vi "Transmitter_SC.vi"() -> ()   [LabVIEW 2022 SP3]
uses:
  <instrlib>/niUSRP/niUSRP Write Tx Data (CDB Cluster).vi
panel:
  in  "Alpha":dbl(slide)=0.17500000000000002 step=0.005 scale=0.0..1.0
  in  "Tab Control":enum32{"USRP Parameters", "Transmission"}(tab)
  in  "USRP ControledParameters 2":T1={"Active Antenna"="TX1", "Gain (dB)"=0.0, "Carrier Frequency"=2400000000.0, "IQ Rate"=2000000.0, "Active Channel"="0"} {"IQ Rate" format="%#_6p"; "Carrier Frequency" format="%#_6p"; "Gain (dB)" format="%#_6f"}
  in  "Device selection":refnum<k15>="RIO0"
  in  "stop":bool
  out "Error out":errorcluster
  in  "Modulation parameter":T2
  out "Bits length":i32
  out "Bits length 2":i32
  out "Frame Duration":dbl format="%#_6p"
  out "Coerced Parameters":T3={"IQ Rate"=100000.0, "Carrier  Freq."=100000.0, "Gain"=0.0} {"Gain" format="%#_6f"; "Carrier  Freq." format="%#_6p"; "IQ Rate" format="%#_6p"}
  out "Transmitted Waveform":cluster{"t0":dbl, "dt":dbl, "Y":dbl[]}(graph)
  in  "Message 2":string="ptua. At vero eos et accusam et justo duo dolores et ea rebum. Stet clita kasd gubergren, no sea takimata sanctus est Lorem ipsum dolor sit amet. Lore"
  in  "Message 1":string="Lorem ipsum dolor sit amet, consetetur sadipscing elitr, sed diam nonumy eirmod tempor invidunt ut labore et dolore magna aliquyam erat, sed diam volu"
  in  "error in (no error)":errorcluster
  # "OFDM Superposition Coded Transmitter"
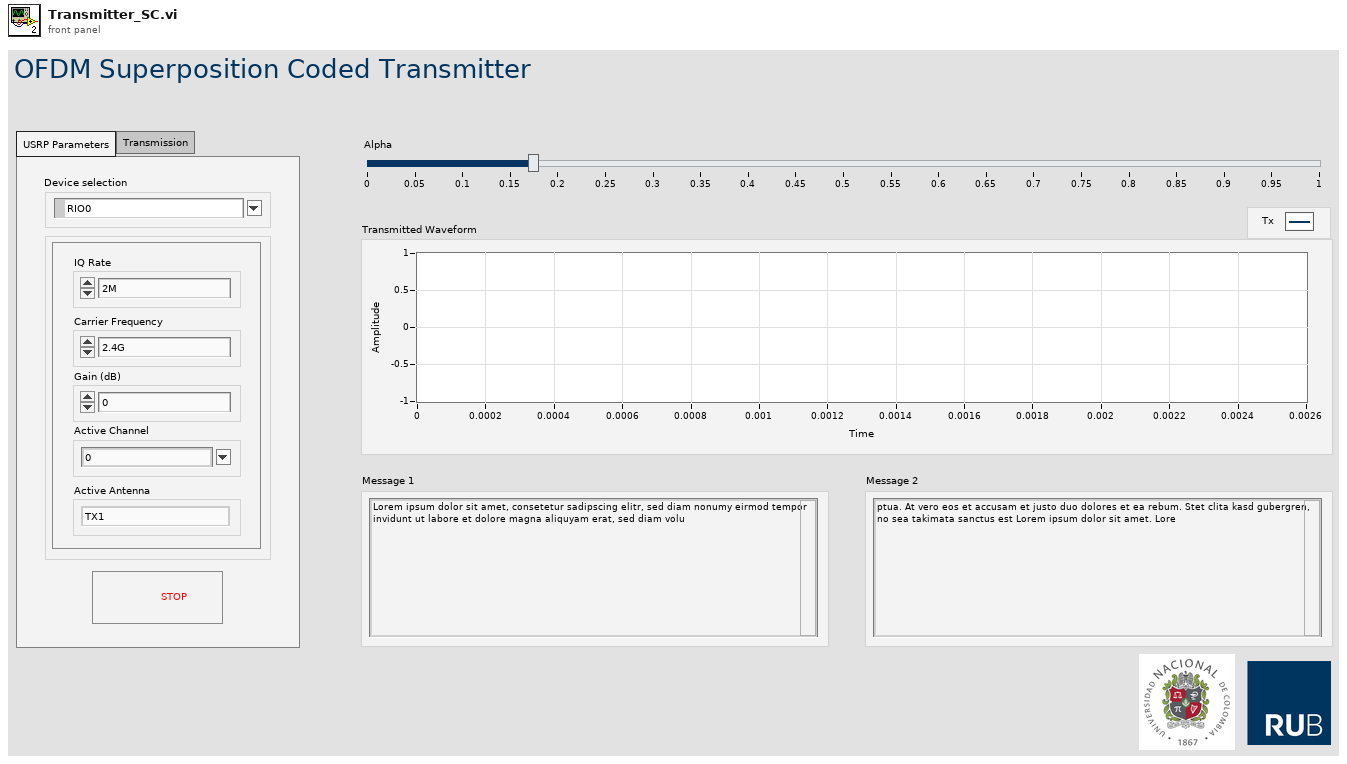
[diagram p1: front panel]
types:
  T1 = cluster{"Active Antenna":string, "Gain (dB)":dbl, "Carrier Frequency":dbl, "IQ Rate":dbl, "Active Channel":string}
  T2 = cluster{"Modulation type":enum16{"QPSK(4QAM)", "64QAM", "16QAM", "BPSK"}, "BCC rate (k/n)":enum16{"1/2", "2/3", "3/4"}}
  T3 = cluster{"IQ Rate":dbl, "Carrier  Freq.":dbl, "Gain":dbl}
  T4 = cluster{"coerced IQ rate":dbl, "coerced carrier frequency":dbl, "coerced gain":dbl}
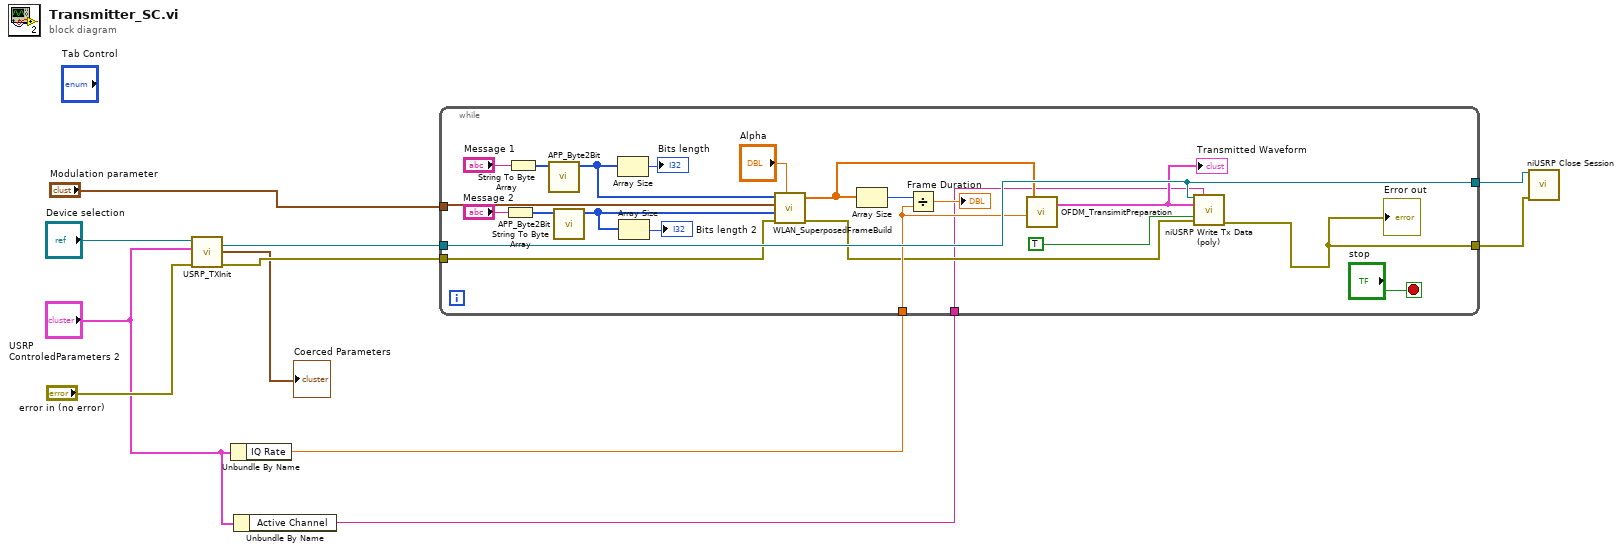
[diagram p0: block diagram]
diagram:
  n1 = call "USRP_TXInit.vi"("device names"="Device selection", "USRP ControledParameters"="USRP ControledParameters 2", "error in (no error)"="error in (no error)") -> ("session handle out"=w10:refnum<k15>, "USRP CoercedParamters"=→"Coerced Parameters":T4, "error out"=w8:errorcluster)  [unwired: 5 in]
  n2 = Unbundle By Name("USRP ControledParameters 2") -> ("IQ Rate"=w7:dbl)
  n3 = Unbundle By Name("USRP ControledParameters 2") -> ("Active Channel"=w1:string)
  n4 = while {
    tunnel: w10 -> [w28]
    tunnel: "Modulation parameter" -> [w20]
    tunnel: w8 -> [w19]
    tunnel: w7 -> [w26]
    tunnel: [w28] -> w6
    tunnel: [w14] -> w5
    tunnel: w1 -> [w12]
    stop <- "stop" stop-if-true
    n5 = String To Byte Array(string="Message 2") -> (unsigned byte array=w22:u8[])
    n6 = String To Byte Array(string="Message 1") -> (unsigned byte array=w24:u8[])
    n7 = call "APP_Byte2Bit.vi"("input byte stream"=w24) -> ("output bit stream"=w16:i8[])  [unwired: 10 in]
    n8 = call "APP_Byte2Bit.vi"("input byte stream"=w22) -> ("output bit stream"=w21:i8[])  [unwired: 10 in]
    n9 = Array Size(array=w16) -> (size(s)=→"Bits length":i32)
    n10 = Array Size(array=w21) -> (size(s)=→"Bits length 2":i32)
    n11 = call "WLAN_SuperposedFrameBuild.vi"("Alpha"="Alpha", "error in (no error)"=w19, "data in 2"=w21, "Modulation parameter"=w20, "data in"=w16) -> ("error out"=w18:errorcluster, "output array"=w17:cdb[])  [unwired: 5 in]
    n12 = Array Size(array=w17) -> (size(s)=w31:i32)
    n13 = Divide(x=w31, y=w26) -> (x/y=→"Frame Duration":dbl)
    n14 = call "OFDM_TransimitPreparation.vi"("IQ rate"=w26, "array"=w17) -> ("output cluster"=w15:cluster{"t0":dbl, "dt":dbl, "Y":cdb[]})  [unwired: 9 in]
    "Transmitted Waveform" <- w15
    n15 = call-poly <instrlib>:"niUSRP Write Tx Data (poly).vi"("session handle"=w28, "channel list"=w12, "data"=w15, "end of data?"=TRUE, "error in (no error)"=w18) -> ("error out"=w14:errorcluster)  [unwired: 9 in, 1 out]
    "Error out" <- w14
  }
  n16 = call <instrlib>:"niUSRP Close Session.vi"("session handle"=w6, "error in (no error)"=w5) -> ()  [unwired: 13 in, 1 out]
